vi "Teleop.vi"(10 "Match Info":T1={"Autonomous Elapsed Seconds"=0.0, "TeleOp Elapsed Seconds"=0.0, "Disabled Elapsed Seconds"=0.0, "Visited Autonomous"=FALSE, "Visited TeleOp"=FALSE, "Visited Disabled"=FALSE, "Autonomous Settings"={"Autonomous Style"=enum."Independent", "VI Refnum"=refnum}}, 11 "Call Context":T2) -> ()   [LabVIEW 2017]
doc: "This VI is called for each TeleOp packet received from the DS where the robot is not disabled. It is often used to read from the joysticks and update I/O or to update setpoints for timed control loops. It should complete and return within 20 milliseconds or it may miss DS packets."
uses:
  <vilib>/Rock Robotics/WPI/DriverStation/WPI_DriverStationDerivedRobotMode.ctl
  <vilib>/Rock Robotics/WPI/DriverStation/WPI_DriverStationMatch Info.ctl
  <vilib>/Rock Robotics/WPI/ThirdParty/Phoenix-LabVIEW/Motor Controller/Controls/CTRE_Phoenix_MotorControl_ControlMode.ctl
  <vilib>/Rock Robotics/WPI/Utilities/WPI_GetSetVariantRefNum.vi
  <vilib>/Rock Robotics/Network Tables/NT Write Numeric Array.vi
  <vilib>/Rock Robotics/Network Tables/NT Read Boolean.vi
  <vilib>/Rock Robotics/Network Tables/NT Read String.vi
  <vilib>/Rock Robotics/Network Tables/NT Write Boolean.vi
  <vilib>/Rock Robotics/Network Tables/NT Read Number.vi
  <vilib>/Rock Robotics/Network Tables/NT Write Boolean Array.vi
  <vilib>/Rock Robotics/Network Tables/NT Write Number.vi
  <vilib>/Rock Robotics/WPI/ThirdParty/Phoenix-LabVIEW/Motor Controller/Get/CTRE_Phoenix_MotorController_GetQuadratureData.vi
panel:
  in  "Invert?":bool
  in  "PhaseSensor":bool
  out "Sensor Pos":i32=1
  out "Sensor Velocity":i32=1
  out "Gamepad output":dbl=1.0 format="%.2f"
  out "Drive Style Selection":string
  out "Sample Slider 0":dbl(slide) scale=0.0..5.0
  out "Sample Boolean 1":bool
  out "Sample Boolean 0":bool
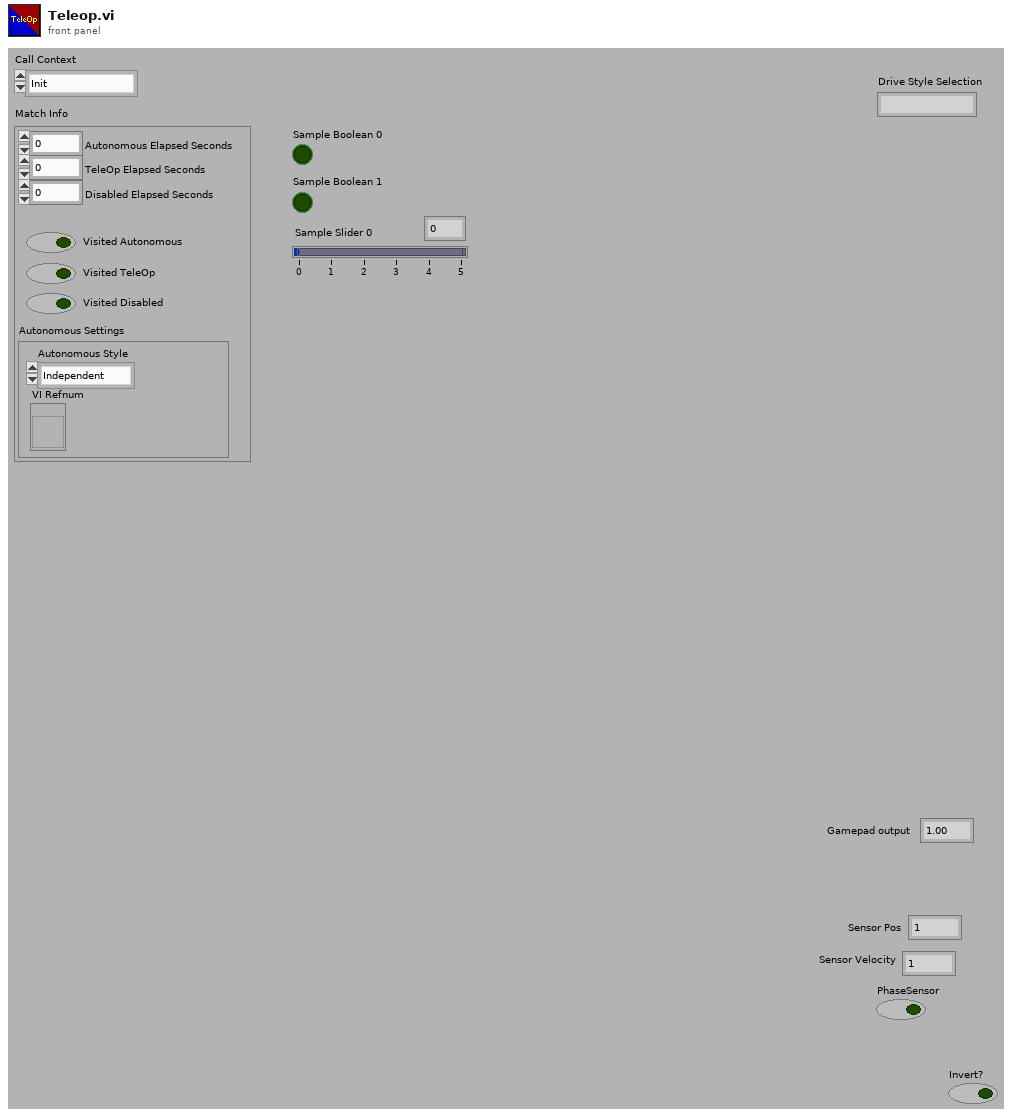
[diagram p1: front panel]
types:
  T1 = typedef "WPI_DriverStationMatch Info.ctl" = cluster{"Autonomous Elapsed Seconds":dbl, "TeleOp Elapsed Seconds":dbl, "Disabled Elapsed Seconds":dbl, "Visited Autonomous":bool, "Visited TeleOp":bool, "Visited Disabled":bool, "Autonomous Settings":cluster{"Autonomous Style":enum16{"Iterative", "Independent"}, "VI Refnum":refnum<vi>}}
  T2 = typedef "WPI_DriverStationDerivedRobotMode.ctl" = enum16{"Init", "Execute", "Stop"}
  T3 = typedef "CTRE_Phoenix_MotorControl_ControlMode.ctl" = u16
  T4 = typedef "WPI_SwitchDevRef.ctl" = cluster{"DevStatus":errorcluster, "DIO Channel":T5, "CntIndex":T6, "Normally Closed":bool}
  T5 = typedef "FPGA_DIOChannel.ctl" = enum8{"DIO 0", "DIO 1", "DIO 2", "DIO 3", "DIO 4", "DIO 5", "DIO 6", "DIO 7", "DIO 8", "DIO 9", "DIO MXP 0", "DIO MXP 1", "DIO MXP 2", "DIO MXP 3", "DIO MXP 4", "DIO MXP 5", "DIO MXP 6", "DIO MXP 7", "DIO MXP 8", "DIO MXP 9", "DIO MXP 10", "DIO MXP 11", "DIO MXP 12", "DIO MXP 13", "DIO MXP 14", "DIO MXP 15", "SPI Port CS1", "SPI Port CS2", "SPI Port CS3", "SPI Port MISO", "SPI Port MOSI", "Invalid"}
  T6 = typedef "FPGA_CounterCtrSystemIndex.ctl" = enum8{"Ctr 0", "Ctr 1", "Ctr 2", "Ctr 3", "Ctr 4", "Ctr 5", "Ctr 6", "Ctr 7", "Invalid"}
  T7 = typedef "WPI_JoystickDevRef.ctl" = cluster{"Device":T8}
  T8 = typedef "WPI_JoystickDeviceEnum.ctl" = enum16{"USB 0", "USB 1", "USB 2", "USB 3", "USB 4", "USB 5"}
  T9 = cluster{"Buttons[0]":bool, "Buttons[1]":bool, "Buttons[2]":bool, "Buttons[3]":bool, "Buttons[4]":bool, "Buttons[5]":bool, "Buttons[6]":bool, "Buttons[7]":bool, "Buttons[8]":bool}
  T10 = cluster{"Axes[0]":dbl, "Axes[1]":dbl, "Axes[2]":dbl, "Axes[3]":dbl, "Axes[4]":dbl, "Axes[5]":dbl, "Axes[6]":dbl, "Axes[7]":dbl, "Axes[8]":dbl}
  T11 = typedef "WPI_MotorControlDeviceRef.ctl" = cluster{"DeviceStatus":errorcluster, "Type":T12, "PWM":cluster{"PWM Channel":T13, "DeadBand":T14}, "CAN":cluster{"Device Number":u8, "SetOutput VI Ref":variant, "GetOutput VI Ref":variant, "Enable VI Ref":variant, "Disable VI Ref":variant, "Data":variant}, "Invert":bool, "DIO PWM":cluster{"PWM \"Enable\" Channel":T13, "DIOChannel":T5, "PWM Rate":dbl}}
  T12 = typedef "WPI_MotorControlType.ctl" = enum16{"PWM", "CAN", "DIO PWM"}
  T13 = typedef "FPGA_DIOPWMChannel.ctl" = enum8{"PWM 0", "PWM 1", "PWM 2", "PWM 3", "PWM 4", "PWM 5", "PWM 6", "PWM 7", "PWM 8", "PWM 9", "PWM MXP 0", "PWM MXP 1", "PWM MXP 2", "PWM MXP 3", "PWM MXP 4", "PWM MXP 5", "PWM MXP 6", "PWM MXP 7", "PWM MXP 8", "PWM MXP 9", "Invalid"}
  T14 = typedef "WPI_PWMDeadband.ctl" = cluster{"Name":string, "maxPositivePwm":i32, "minPositivePwm":i32, "centerPwm":i32, "maxNegativePwm":i32, "minNegativePwm":i32, "angularRange":u16}
  T15 = typedef "WPI_RobotDriveDevRef.ctl" = cluster{"DevStatus":errorcluster, "Motors[]":T11[], "Square Inputs":bool, "Max Output":dbl}
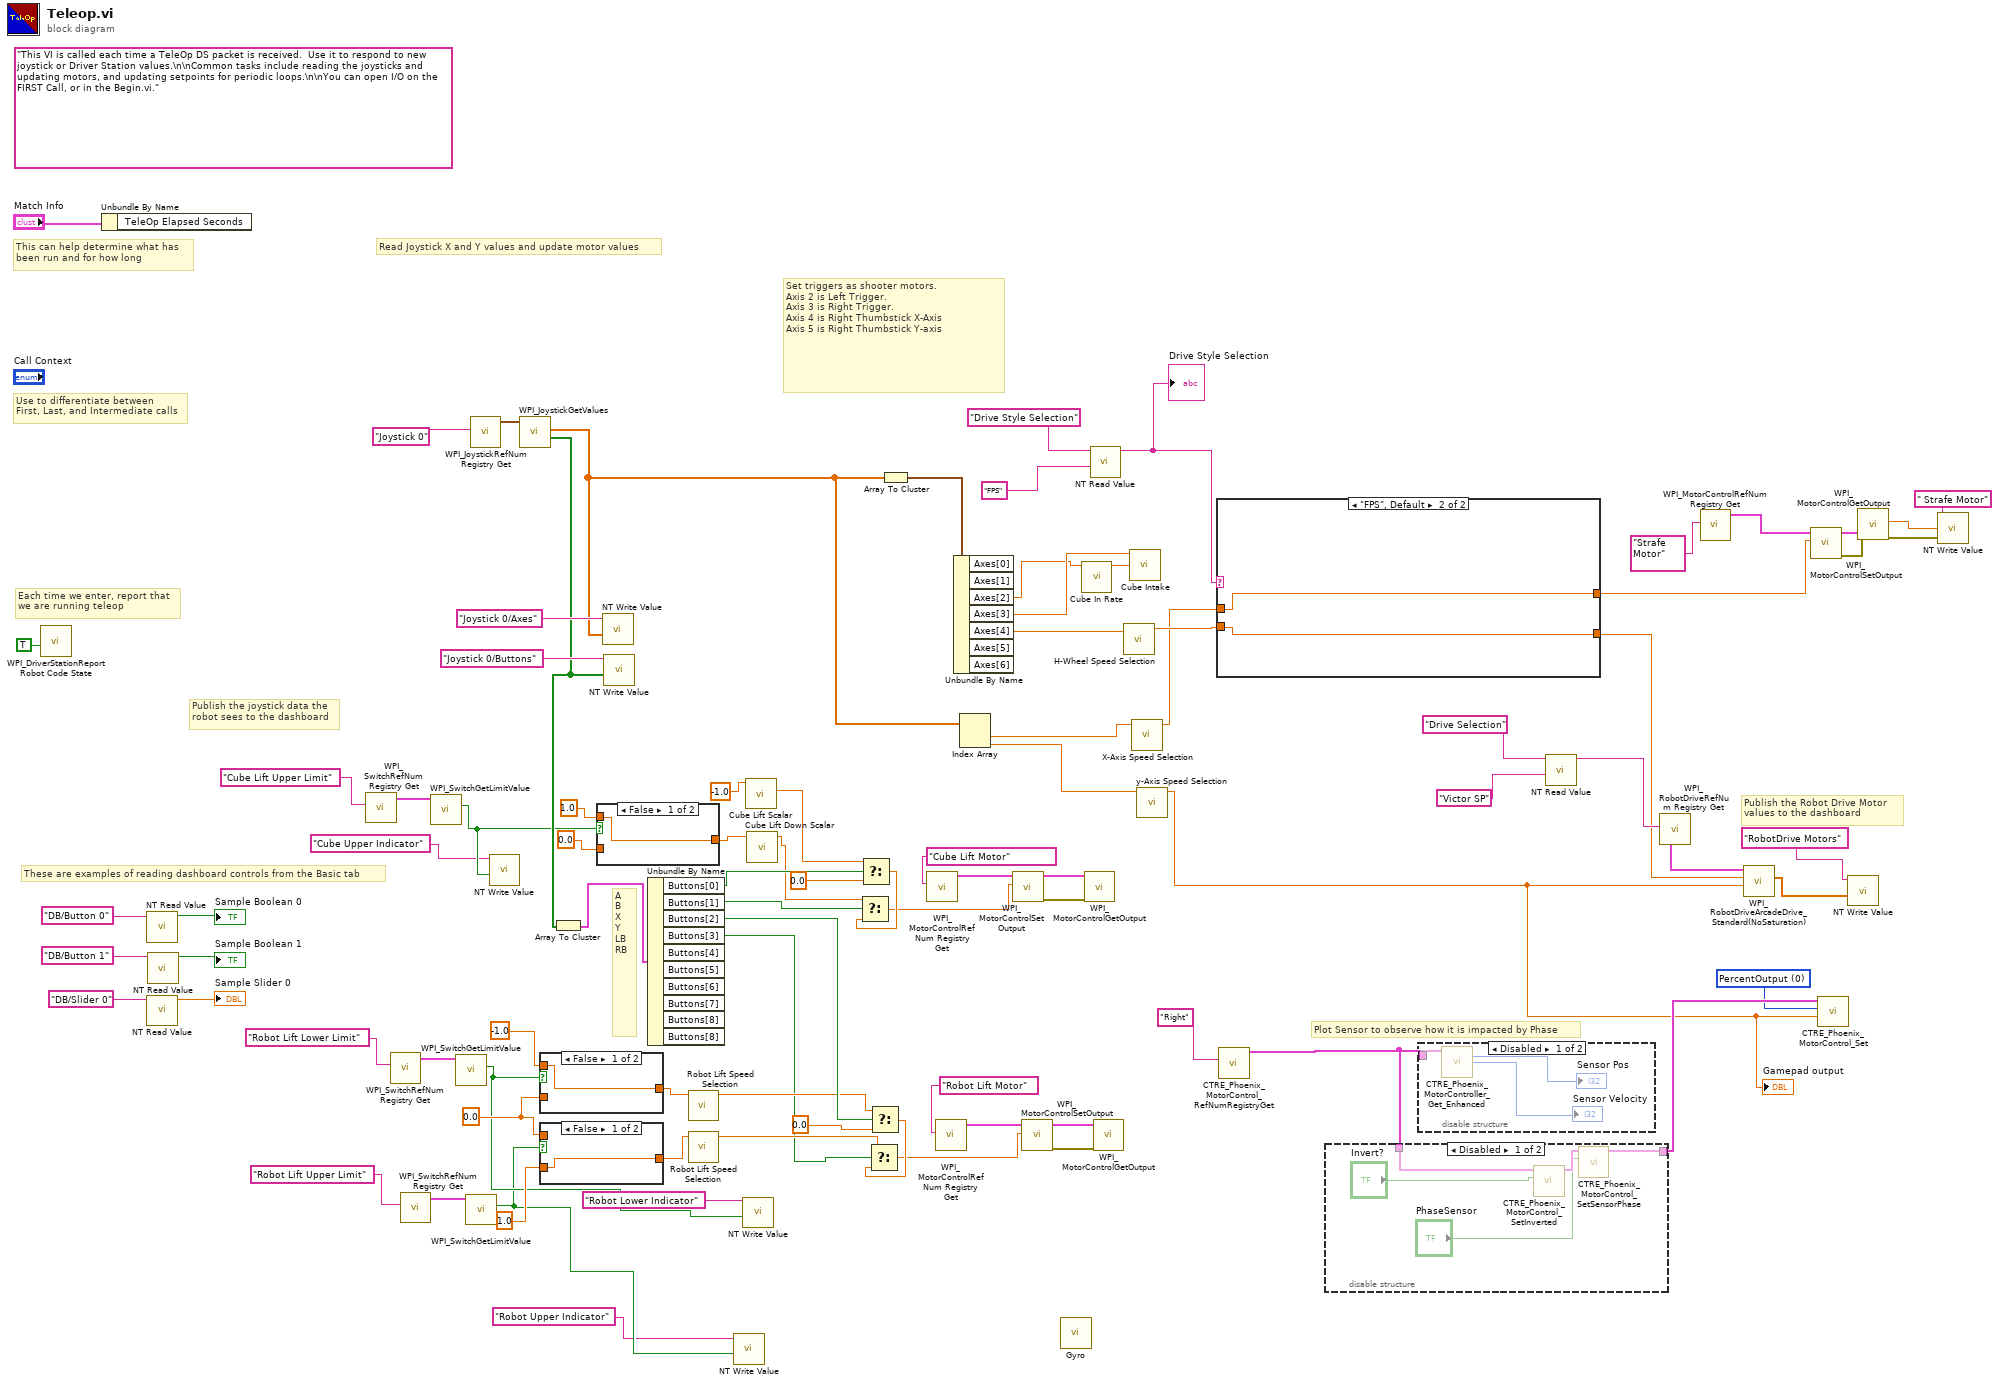
[diagram p0: block diagram]
diagram:
  w14 = 0.0
  w22 = T3 0 items=["PercentOutput"=0, "Position"=1, "Velocity"=2, "Current"=3, "Follower"=5, "MotionProfile"=6, "MotionMagic"=7, "MotionMagicArc"=8, "MotionProfileArc"=10, "Disabled"=15] ("Control Mode")
  (unwired) "This VI is called each time a TeleOp DS packet is received.  Use it to respond to new joystick or Driver Station values.\n\nCommon tasks include reading the joysticks and updating motors, and updating setpoints for periodic loops.\n\nYou can open I/O on the FIRST Call, or in the Begin.vi."
  # "Plot Sensor to observe how it is impacted by Phase"
  # "Publish the Robot Drive Motor\nvalues to the dashboard"
  # "Set triggers as shooter motors.  \nAxis 2 is Left Trigger.  \nAxis 3 is Right Trigger.\nAxis 4 is Right Thumbstick X-Axis\nAxis 5 is Right Thumbstick Y-axis"
  # "A\nB\nX\nY\nLB\nRB"
  # "These are examples of reading dashboard controls from the Basic tab"
  # "Publish the joystick data the\nrobot sees to the dashboard"
  # "Each time we enter, report that\nwe are running teleop"
  # "Use to differentiate between\nFirst, Last, and Intermediate calls"
  # "This can help determine what has\nbeen run and for how long"
  # "Read Joystick X and Y values and update motor values"
  n1 = call <vilib>:"WPI_DriverStationReport Robot Code State.vi"("TeleOp"=TRUE ("Autonomous")) -> ()  [unwired: 10 in, 1 out]
  n2 = Unbundle By Name("Match Info") -> ()  [unwired: 1 out]
  n3 = call-poly <vilib>:"NT Read Value.vi"("Name"="DB/Button 0" ("refnum name")) -> ("Boolean"=→"Sample Boolean 0":bool)  [unwired: 9 in, 1 out]
  n4 = call-poly <vilib>:"NT Read Value.vi"("Name"="DB/Slider 0" ("refnum name")) -> ("Numeric"=→"Sample Slider 0":dbl)  [unwired: 9 in, 1 out]
  n5 = call-poly <vilib>:"NT Read Value.vi"("Name"="DB/Button 1" ("refnum name")) -> ("Boolean"=→"Sample Boolean 1":bool)  [unwired: 9 in, 1 out]
  n6 = call <vilib>:"WPI_SwitchRefNum Registry Get.vi"("refnum name"="Cube Lift Upper Limit") -> ("SwitchDevRef"=w10:T4)  [unwired: 9 in, 1 out]
  n7 = call <vilib>:"WPI_SwitchRefNum Registry Get.vi"("refnum name"="Robot Lift Lower Limit") -> ("SwitchDevRef"=w18:T4)  [unwired: 9 in, 1 out]
  n8 = call <vilib>:"WPI_SwitchRefNum Registry Get.vi"("refnum name"="Robot Lift Upper Limit") -> ("SwitchDevRef"=w19:T4)  [unwired: 9 in, 1 out]
  n9 = call <vilib>:"WPI_SwitchGetLimitValue.vi"("SwitchDevRef"=w10) -> ("Switch Pressed"=w2:bool)  [unwired: 8 in, 2 out]
  n10 = call <vilib>:"WPI_SwitchGetLimitValue.vi"("SwitchDevRef"=w18) -> ("Switch Pressed"=w6:bool)  [unwired: 8 in, 2 out]
  n11 = call <vilib>:"WPI_SwitchGetLimitValue.vi"("SwitchDevRef"=w19) -> ("Switch Pressed"=w5:bool)  [unwired: 8 in, 2 out]
  n12 = call <vilib>:"WPI_JoystickRefNum Registry Get.vi"("refnum name"="Joystick 0") -> ("JoystickDevRef"=w88:T7)  [unwired: 1 in, 9 out]
  n13 = call-poly <vilib>:"NT Write Value.vi"("Boolean"=w2, "Name"="Cube Upper Indicator") -> ()  [unwired: 9 in, 1 out]
  n14 = call <vilib>:"WPI_JoystickGetValues.vi"("JoystickDevRef"=w88) -> ("Buttons"=w78:bool[], "Axes"=w44:dbl[])  [unwired: 6 in, 3 out]
  n15 = case shown="False" w6 {
    tunnel: w14 -> [_ w92]
    tunnel: [w91 w92] -> w12
    tunnel: -1.0 -> [w91 _]
    frame False {
    }
    frame True {
    }
  }
  n16 = case shown="False" w5 {
    tunnel: 1.0 -> [w93 _]
    tunnel: [w93 w94] -> w15
    tunnel: w14 -> [_ w94]
    frame False {
    }
    frame True {
    }
  }
  n17 = Array To Cluster(array=w78) -> (cluster=w71:T9)
  n18 = case shown="False" w2 {
    tunnel: 0.0 -> [_ w96]
    tunnel: [w95 w96] -> w7
    tunnel: 1.0 -> [w95 _]
    frame False {
    }
    frame True {
    }
  }
  n19 = call-poly <vilib>:"NT Write Value.vi"("Numeric Array"=w44, "Name"="Joystick 0/Axes") -> ()  [unwired: 9 in, 1 out]
  n20 = call-poly <vilib>:"NT Write Value.vi"("Boolean Array"=w78, "Name"="Joystick 0/Buttons") -> ()  [unwired: 9 in, 1 out]
  n21 = Unbundle By Name(w71) -> ("Buttons[0]"=w69:bool, "Buttons[1]"=w70:bool, "Buttons[2]"=w58:bool, "Buttons[3]"=w52:bool)  [unwired: 6 out]
  n22 = call "Robot Lift Speed Selection.vi"("upper limit in"=w12) -> ("upper limit out"=w56:dbl)  [unwired: 10 in]
  n23 = call "Robot Lift Speed Selection.vi"("upper limit in"=w15) -> ("upper limit out"=w55:dbl)  [unwired: 10 in]
  n24 = call-poly <vilib>:"NT Write Value.vi"("Boolean"=w5, "Name"="Robot Upper Indicator") -> ()  [unwired: 9 in, 1 out]
  n25 = call-poly <vilib>:"NT Write Value.vi"("Boolean"=w6, "Name"="Robot Lower Indicator") -> ()  [unwired: 9 in, 1 out]
  n26 = call "Cube Lift Scalar.vi"("upper limit in"=-1.0) -> ("upper limit out"=w54:dbl)  [unwired: 10 in]
  n27 = call "Cube Lift Down Scalar.vi"("upper limit in"=w7) -> ("upper limit out"=w57:dbl)  [unwired: 10 in]
  n28 = Select(t=w54, s=w69, f=0.0) -> (s? t:f=w67:dbl)
  n29 = Select(t=w57, s=w70, f=w67) -> (s? t:f=w66:dbl)
  n30 = Select(t=w56, s=w58, f=0.0) -> (s? t:f=w60:dbl)
  n31 = Select(t=w55, s=w52, f=w60) -> (s? t:f=w59:dbl)
  n32 = Array To Cluster(array=w44) -> (cluster=w77:T10)
  n33 = call <vilib>:"WPI_MotorControlRefNum Registry Get.vi"("refnum name"="Cube Lift Motor") -> ("MotorControlDevRef"=w73:T11)  [unwired: 9 in, 1 out]
  n34 = call <vilib>:"WPI_MotorControlRefNum Registry Get.vi"("refnum name"="Robot Lift Motor") -> ("MotorControlDevRef"=w63:T11)  [unwired: 9 in, 1 out]
  n35 = Unbundle By Name(w77) -> ("Axes[2]"=w51:dbl, "Axes[3]"=w76:dbl, "Axes[4]"=w49:dbl)  [unwired: 4 out]
  n36 = Index Array "Index Array"(array=w44) -> (element #1=w28:dbl, element #2=w26:dbl)  [unwired: 2 in]
  n37 = call <vilib>:"WPI_MotorControlSetOutput.vi"("Output"=w66, "MotorControlDevRef"=w73) -> ("error out"=w75:errorcluster, "MotorControlDevRef"=w74:T11)  [unwired: 7 in, 1 out]
  n38 = call <vilib>:"WPI_MotorControlSetOutput.vi"("Output"=w59, "MotorControlDevRef"=w63) -> ("error out"=w65:errorcluster, "MotorControlDevRef"=w64:T11)  [unwired: 7 in, 1 out]
  n39 = call "Gyro.vi"() -> ()  [unwired: 12 in]
  n40 = call "Cube In Rate.vi"("upper limit in"=w51) -> ("upper limit out"=w50:dbl)  [unwired: 10 in]
  n41 = call <vilib>:"WPI_MotorControlGetOutput.vi"("error in"=w75, "MotorControlDevRef"=w74) -> ()  [unwired: 7 in, 3 out]
  n42 = call-poly <vilib>:"NT Read Value.vi"("Default Value"="FPS", "Name"="Drive Style Selection") -> ("String"=w45:string)  [unwired: 8 in, 1 out]
  "Drive Style Selection" <- w45
  n43 = call <vilib>:"WPI_MotorControlGetOutput.vi"("error in"=w65, "MotorControlDevRef"=w64) -> ()  [unwired: 7 in, 3 out]
  n44 = call "H-Wheel Speed Selection.vi"("upper limit in"=w49) -> ("upper limit out"=w48:dbl)  [unwired: 10 in]
  n45 = call "Cube Intake.vi"("Axes[2]"=w50, "Axes[3]"=w76) -> ()  [unwired: 10 in]
  n46 = call "X-Axis Speed Selection.vi"("upper limit in"=w28) -> ("upper limit out"=w27:dbl)  [unwired: 10 in]
  n47 = call "y-Axis Speed Selection.vi"("upper limit in"=w26) -> ("upper limit out"=w21:dbl)  [unwired: 10 in]
  "Gamepad output" <- w21
  n48 = case shown="\"FPS\", Default" w45 {
    tunnel: w48 -> [w97 w100]
    tunnel: [w98 w100] -> w29
    tunnel: w27 -> [w98 w99]
    tunnel: [w97 w99] -> w36
    frame "Arcade" {
    }
    frame "FPS", Default {
    }
  }
  n49 = call <vilib>:"CTRE_Phoenix_MotorControl_RefNumRegistryGet.vi"("refnum name"="Right") -> ("PhoenixMotorControlDevRef"=w24:T11)  [unwired: 9 in, 1 out]
  n50 = disable-structure shown="Disabled" {
    disable-tunnel: w24 -> [w102 _]
    disable-tunnel: [w101 _] -> w23
    frame Disabled {
      n51 = call <vilib>:"CTRE_Phoenix_MotorControl_SetInverted.vi"("Invert?"="Invert?", "PhoenixMotorControlDevRef"=w102) -> ("PhoenixMotorControlDevRef"=w105:T11)  [unwired: 8 in, 1 out]
      n52 = call <vilib>:"CTRE_Phoenix_MotorControl_SetSensorPhase.vi"("PhaseSensor"="PhaseSensor", "PhoenixMotorControlDevRef"=w105) -> ("PhoenixMotorControlDevRef"=w101:T11)  [unwired: 8 in, 1 out]
    }
    frame Enabled {
    }
  }
  n53 = disable-structure shown="Disabled" {
    disable-tunnel: w24 -> [w106 _]
    frame Disabled {
      n54 = call-poly <vilib>:"CTRE_Phoenix_MotorController_Get_Enhanced.vi"("PhoenixMotorControlDevRef"=w106) -> ("Quadrature Position"=→"Sensor Pos":i32, "Quadrature Velocity"=→"Sensor Velocity":i32)  [unwired: 11 in, 2 out]
    }
    frame Enabled {
    }
  }
  n55 = call-poly <vilib>:"NT Read Value.vi"("Default Value"="Victor SP", "Name"="Drive Selection") -> ("String"=w30:string)  [unwired: 8 in, 1 out]
  n56 = call <vilib>:"WPI_RobotDriveRefNum Registry Get.vi"("refnum name"=w30) -> ("RobotDriveDevRef"=w35:T15)  [unwired: 1 in, 9 out]
  n57 = call <vilib>:"WPI_MotorControlRefNum Registry Get.vi"("refnum name"="Strafe Motor") -> ("MotorControlDevRef"=w42:T11)  [unwired: 9 in, 1 out]
  n58 = call <vilib>:"WPI_RobotDriveArcadeDrive_Standard(NoSaturation).vi"("Y axis value"=w21, "X axis value"=w29, "RobotDriveDevRef"=w35) -> ("Motor Values"=w34:dbl[])  [unwired: 1 in, 7 out]
  n59 = call <vilib>:"WPI_MotorControlSetOutput.vi"("Output"=w36, "MotorControlDevRef"=w42) -> ("error out"=w40:errorcluster, "MotorControlDevRef"=w41:T11)  [unwired: 7 in, 1 out]
  n60 = call <vilib>:"CTRE_Phoenix_MotorControl_Set.vi"("Output"=w21, "Control Mode"=w22, "PhoenixMotorControlDevRef"=w23) -> ()  [unwired: 7 in, 2 out]
  n61 = call-poly <vilib>:"NT Write Value.vi"("Numeric Array"=w34, "Name"="RobotDrive Motors") -> ()  [unwired: 9 in, 1 out]
  n62 = call <vilib>:"WPI_MotorControlGetOutput.vi"("error in"=w40, "MotorControlDevRef"=w41) -> ("error out"=w38:errorcluster, "Output"=w37:dbl)  [unwired: 7 in, 1 out]
  n63 = call-poly <vilib>:"NT Write Value.vi"("error in"=w38, "Numeric"=w37, "Name"=" Strafe Motor") -> ()  [unwired: 8 in, 1 out]
